vi "SIMDMM_subUserDefinedVals.vi"(0 "t0":dbl format="%0.2f", 1 "Next Value":bool, 3 "Mode":i32, 5 "dt":dbl=0.01 format="%0.2f", 7 "error in (no error)":errorcluster, 9 "Array":dbl[][](array[numeric]) format="%0.2f", 11 "Signal Name":string, 12 "Cycle through Values":bool, 13 "Repeat":bool, 14 "Reset":bool) -> (4 "Signal":dynamicdata(graph), 8 "error out":errorcluster, 10 "Data Valid":bool)   [LabVIEW 2019]
uses:
  SIMDMM_ex_WaveformAttribsPlus.ctl
panel:
  in  "Express Atttributes":T1 {"dX" format="%.2f"; "X0" format="%<%X\n%x>T"; "Timestamp" format="%<%X\n%x>T"; "Start Timestamp" format="%<%X\n%x>T"}
  in  "Index for To":i32
  in  "Index of Array":i32
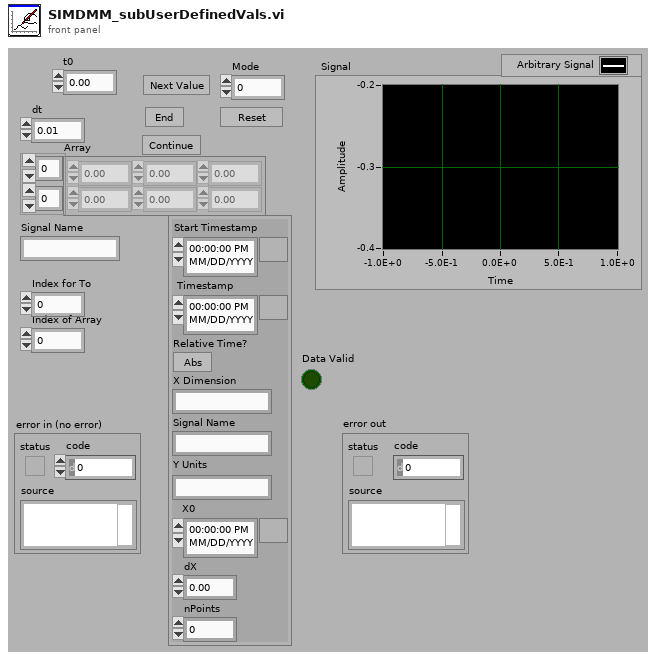
[diagram p1: front panel]
types:
  T1 = typedef "SIMDMM_ex_WaveformAttribsPlus.ctl" = cluster{"Start Timestamp":timestamp, "Timestamp":timestamp, "Relative Time?":bool, "X Dimension":string, "Signal Name":string, "Y Units":string, "X0":timestamp, "dX":dbl, "nPoints":i32}
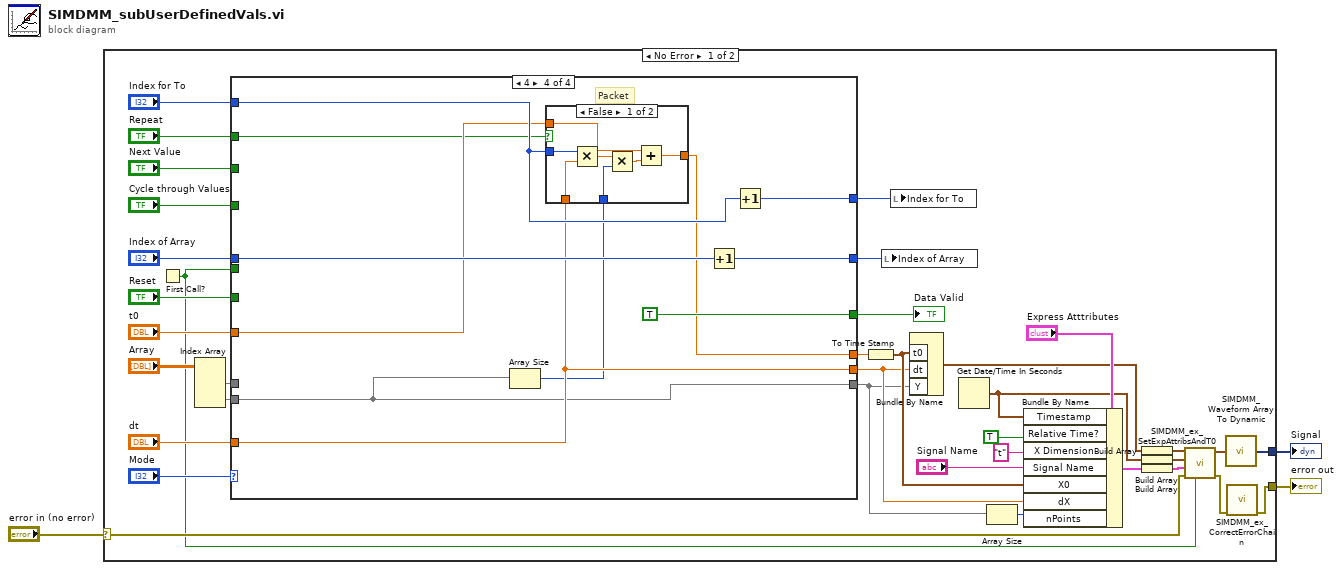
[diagram p0: block diagram]
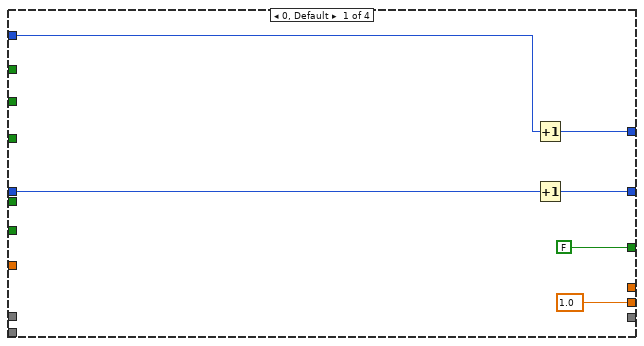
[diagram p2: hidden frame]
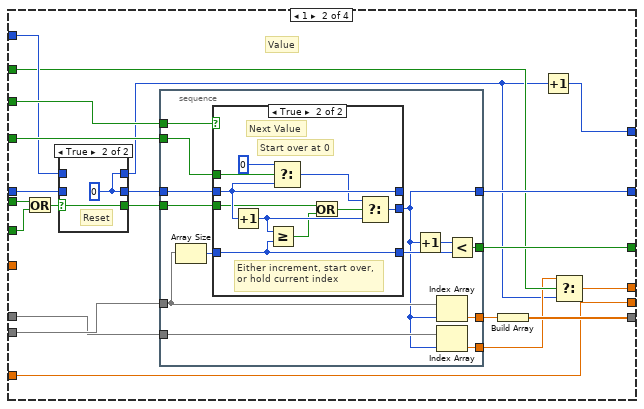
[diagram p3: hidden frame]
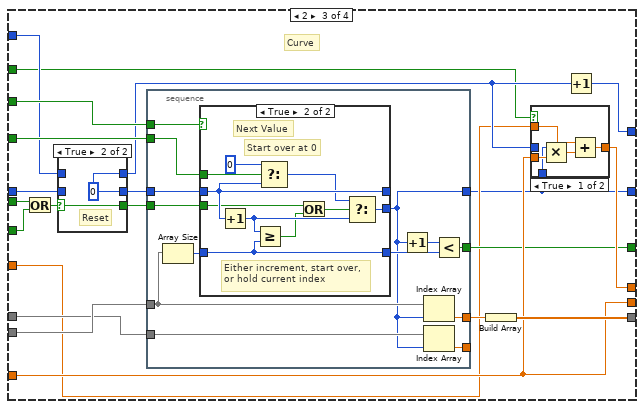
[diagram p6: hidden frame]
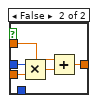
[diagram p7: hidden frame]
diagram:
  n1 = case shown="No Error" "error in (no error)" {
    selector: "error in (no error)" -> [w13 w177]
    tunnel: [w37 _] -> w3
    tunnel: [w4 w177] -> w1
    frame No Error {
      n2 = First Call?() -> (First Call?: T/F=w12:bool)
      n3 = Index Array(array="Array") -> (element #1=w28:dbl[], element #2=w29:dbl[])  [unwired: 4 in]
      n4 = case shown="4" "Mode" {
        tunnel: "t0" -> [_ _ w100 w162]
        tunnel: "dt" -> [_ w51 w106 w160]
        tunnel: w29 -> [_ w62 w113 w159]
        tunnel: [w42 w52 w99 w166] -> w31
        tunnel: "Index of Array" -> [w45 w61 w112 w168]
        tunnel: "Reset" -> [_ w60 w111 _]
        tunnel: "Cycle through Values" -> [_ w59 w110 _]
        tunnel: "Next Value" -> [_ w58 w109 _]
        tunnel: [FALSE w53 w101 TRUE] -> w30
        tunnel: [1.0 ("dt") w51 w106 w160] -> w8
        tunnel: [_ w57 w108 w159] -> w6
        tunnel: w28 -> [_ w56 w107 _]
        tunnel: [_ w47 w105 w163] -> w16
        tunnel: "Repeat" -> [_ w50 w98 w161]
        tunnel: "Index for To" -> [w40 w54 w103 w164]
        tunnel: [w41 w55 w104 w165] -> w25
        tunnel: w12 -> [_ w46 w97 _]
        frame 0, Default {
          n5 = Increment(x=w40) -> (x+1=w41:i32)
          n6 = Increment(x=w45) -> (x+1=w42:i32)
        }
        frame 1 {
          # "Value"
          n7 = Or(x=w46, y=w60) -> (x .or. y?=w65:bool)
          n8 = case shown="True" w65 {
            selector: w65 -> [w68 w71]
            tunnel: w61 -> [w69 _]
            tunnel: [w69 w70] -> w66
            tunnel: [w68 w71] -> w64
            tunnel: w54 -> [w67 _]
            tunnel: [w67 w70] -> w48
            frame False {
            }
            frame True {
              w70 = 0 ("Index")
              # "Reset"
            }
          }
          n9 = stacked-sequence {
            tunnel: w66 -> [w82]
            tunnel: w62 -> [w81]
            tunnel: w59 -> [w80]
            tunnel: [w79] -> w53
            tunnel: [w78] -> w63
            tunnel: [w73] -> w52
            tunnel: w58 -> [w76]
            tunnel: w64 -> [w75]
            tunnel: w56 -> [w74]
            tunnel: [w72] -> w49
            frame #0 {
              n10 = Array Size(array=w81) -> (size(s)=w83:i32)
              n11 = case shown="True" w76 {
                tunnel: w82 -> [w85 w91]
                tunnel: [w85 w91] -> _
                tunnel: [w86 w95] -> w84
                tunnel: w83 -> [w86 w95]
                tunnel: [w85 w94] -> w73
                tunnel: w80 -> [_ w93]
                tunnel: w75 -> [_ w87]
                frame False {
                  # "Same Value"
                }
                frame True {
                  # "Either increment, start over,\nor hold current index"
                  # "Start over at 0"
                  # "Next Value"
                  n12 = Increment(x=w91) -> (x+1=w96:i32)
                  n13 = Greater Or Equal?(x=w96, y=w95) -> (x >= y?=w89:bool)
                  n14 = Select(t=0, s=w93, f=w91) -> (s? t:f=w90:i32)
                  n15 = Or(x=w87, y=w89) -> (x .or. y?=w88:bool)
                  n16 = Select(t=w90, s=w88, f=w96) -> (s? t:f=w94:i32)
                }
              }
              n17 = Increment(x=w73) -> (x+1=w77:i32)
              n18 = Index Array(array=w81, index=w73) -> (element=w78:dbl)
              n19 = Index Array(array=w74, index=w73) -> (element=w72:dbl)
              n20 = Less?(x=w77, y=w84) -> (x < y?=w79:bool)
            }
          }
          n21 = Build Array(w63) -> (w57:dbl[])
          n22 = Increment(x=w48) -> (x+1=w55:i32)
          n23 = Select(t=w49, s=w50, f=w48) -> (s? t:f=w47:dbl)
        }
        frame 2 {
          # "Curve"
          n24 = Or(x=w97, y=w111) -> (x .or. y?=w116:bool)
          n25 = case shown="True" w116 {
            selector: w116 -> [w129 w132]
            tunnel: w112 -> [w130 _]
            tunnel: [w130 w131] -> w117
            tunnel: [w129 w132] -> w115
            tunnel: [w128 w131] -> w102
            tunnel: w103 -> [w128 _]
            frame False {
            }
            frame True {
              w131 = 0 ("Index")
              # "Reset"
            }
          }
          n26 = stacked-sequence {
            tunnel: w117 -> [w143]
            tunnel: w113 -> [w142]
            tunnel: w110 -> [w141]
            tunnel: [w140] -> w101
            tunnel: [w139] -> w114
            tunnel: [w134] -> w99
            tunnel: w109 -> [w137]
            tunnel: w115 -> [w136]
            tunnel: w107 -> [w135]
            tunnel: [w133] -> _
            frame #0 {
              n27 = Array Size(array=w142) -> (size(s)=w144:i32)
              n28 = case shown="True" w137 {
                tunnel: w143 -> [w146 w152]
                tunnel: [w146 w152] -> _
                tunnel: [w147 w156] -> w145
                tunnel: w144 -> [w147 w156]
                tunnel: [w146 w155] -> w134
                tunnel: w141 -> [_ w154]
                tunnel: w136 -> [_ w148]
                frame False {
                  # "Same Value"
                }
                frame True {
                  # "Either increment, start over,\nor hold current index"
                  # "Start over at 0"
                  # "Next Value"
                  n29 = Increment(x=w152) -> (x+1=w157:i32)
                  n30 = Greater Or Equal?(x=w157, y=w156) -> (x >= y?=w150:bool)
                  n31 = Select(t=0, s=w154, f=w152) -> (s? t:f=w151:i32)
                  n32 = Or(x=w148, y=w150) -> (x .or. y?=w149:bool)
                  n33 = Select(t=w151, s=w149, f=w157) -> (s? t:f=w155:i32)
                }
              }
              n34 = Increment(x=w134) -> (x+1=w138:i32)
              n35 = Index Array(array=w142, index=w134) -> (element=w139:dbl)
              n36 = Index Array(array=w135, index=w134) -> (element=w133:dbl)
              n37 = Less?(x=w138, y=w145) -> (x < y?=w140:bool)
            }
          }
          n38 = Build Array(w114) -> (w108:dbl[])
          n39 = case shown="True" w98 {
            tunnel: w102 -> [_ w123]
            tunnel: w100 -> [w120 w125]
            tunnel: w106 -> [w122 w127]
            tunnel: [w119 w124] -> w105
            tunnel: w99 -> [w118 _]
            frame True {
              n40 = Multiply(x=w118, y=w122) -> (x*y=w121:dbl)
              n41 = Add(x=w120, y=w121) -> (x+y=w119:dbl)
            }
            frame False {
              n42 = Multiply(x=w123, y=w127) -> (x*y=w126:dbl)
              n43 = Add(x=w125, y=w126) -> (x+y=w124:dbl)
            }
          }
          n44 = Increment(x=w102) -> (x+1=w104:i32)
        }
        frame 4 {
          # "Packet"
          n45 = Array Size(array=w159) -> (size(s)=w158:i32)
          n46 = case shown="False" w161 {
            tunnel: w164 -> [w175 _]
            tunnel: w162 -> [w172 w176]
            tunnel: [w169 w176] -> w163
            tunnel: w160 -> [w174 _]
            tunnel: w158 -> [w171 _]
            frame False {
              n47 = Multiply(x=w175, y=w174) -> (x*y=w170:dbl)
              n48 = Multiply(x=w170, y=w171) -> (x*y=w173:dbl)
              n49 = Add(x=w172, y=w173) -> (x+y=w169:dbl)
            }
            frame True {
            }
          }
          n50 = Increment(x=w168) -> (x+1=w166:i32)
          n51 = Increment(x=w164) -> (x+1=w165:i32)
        }
      }
      "Data Valid" <- w30
      n52 = To Time Stamp(1:w16) -> (0:w9:timestamp)
      n53 = local write "Index of Array"(w31) -> ()
      n54 = local write "Index for To"(w25) -> ()
      n55 = Bundle By Name("t0"=w9, "dt"=w8, "Y"=w6) -> (w21:waveform(dbl))  [unwired: 1 in]
      n56 = Get Date/Time In Seconds() -> (seconds since 1Jan1904=w14:timestamp)
      n57 = Array Size(array=w6) -> (size(s)=w7:i32)
      n58 = Bundle By Name(cluster="Express Atttributes", "Timestamp"=w14, "Relative Time?"=TRUE ("relative time?"), "X Dimension"="t", "Signal Name"="Signal Name", "X0"=w9, "dX"=w8, "nPoints"=w7) -> (w22:T1)
      n59 = Build Array(w21) -> (w19:waveform(dbl)[])
      n60 = Build Array(w14) -> (w10:timestamp[])
      n61 = Build Array(w22) -> (w11:T1[])
      n62 = call "SIMDMM_ex_SetExpAttribsAndT0.vi"("Latch Origin TS? (T)"=w12, "error in (no error)"=w13, "Express Attributes Plus in"=w11, "Origin Timestamps"=w10, "Signals"=w19) -> ("error out"=w5:errorcluster, "Signals With Attributes"=w18:waveform(dbl)[])  [unwired: 4 in, 1 out]
      n63 = call "SIMDMM_Waveform Array To Dynamic.vi"("Input"=w18) -> ("Output"=w37:dynamicdata)  [unwired: 4 in]
      n64 = call "SIMDMM_ex_CorrectErrorChain.vi"("error in (no error)"=w5) -> ("error out"=w4:errorcluster)  [unwired: 10 in]
    }
    frame Error {
    }
  }
  "Signal" <- w3
  "error out" <- w1
